vi "Estimate Posture from Velocity.vi"(8 "initialize":bool, 9 "dt (s)":dbl=1.0 format="%0.2f", 10 "initial posture":dbl[](array[numeric])=[0.0, 0.0, 0.0], 11 "estimated steering frame velocity":dbl[](array[numeric])=[0.0, 0.0, 0.0]) -> (3 "estimated steering frame posture":dbl[](array[numeric]))   [LabVIEW 2016]
doc: "This VI estimates the posture of a robot by integrating the measured velocity.\n\nThe velocity is a three element array consisting of lateral, forward, and angular velocities relative to the robot's frame of reference.\n\nThe posture is a three element array consiting of the X, Y, and angular position relative to a fixed global frame of reference."
uses:
  <vilib>/Analysis/coordinate.llb/Angle Range (Degree).ctl
  <vilib>/Analysis/coordinate.llb/Angle Units.ctl
  <vilib>/Analysis/coordinate.llb/Wrap Angle (scalar).vi
  <vilib>/Analysis/coordinate.llb/2D Cartesian Coordinate Rotation (Scalar).vi
  <vilib>/ptbypt/NI_PtbyPt.lvlib
  <vilib>/Analysis/NI_AALPro.lvlib
  <vilib>/Analysis/NI_AAL_Angle.lvlib
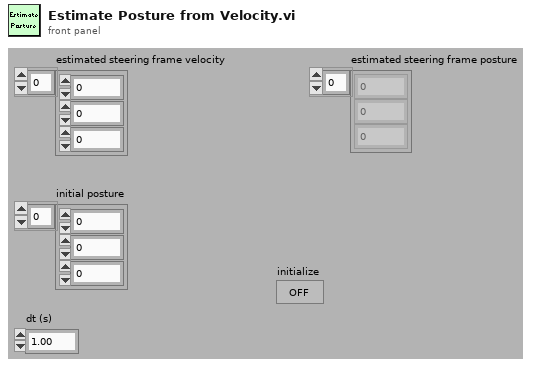
[diagram p1: front panel]
types:
  T1 = typedef "NI_AAL_Angle.lvlib/Angle Units.ctl" = i32
  T2 = typedef "NI_AAL_Angle.lvlib/Angle Range (Degree).ctl" = u16
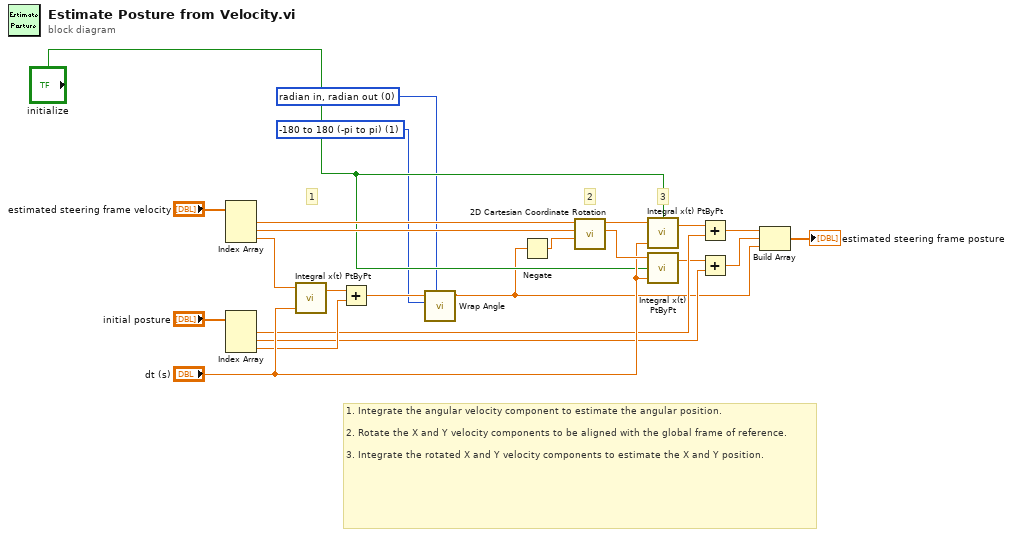
[diagram p0: block diagram]
diagram:
  w1 = T1 0 items=["radian in, radian out", "radian in, degree out", "degree in, degree out", "degree in, radian out"] ("angle units")
  w2 = T2 1 items=["none", "-180 to 180 (-pi to pi)", "0 to 360 (0 to 2pi)"] ("angle range")
  # "3"
  # "2"
  # "1. Integrate the angular velocity component to estimate the angular position.\n\n2. Rotate the X and Y velocity components to be aligned with the global frame of reference.\n\n3. Integrate the rotated X and Y velocity components to estimate the X and Y position."
  # "1"
  n1 = Index Array(array="estimated steering frame velocity") -> (element #1=w19:dbl, element #2=w18:dbl, element #3=w22:dbl)  [unwired: 3 in]
  n2 = Index Array(array="initial posture") -> (element #1=w11:dbl, element #2=w8:dbl, element #3=w13:dbl)  [unwired: 3 in]
  n3 = call <vilib>:"Integral x(t) PtByPt.vi"("dt"="dt (s)", "x"=w22) -> ("integral x(t)"=w12:dbl)  [unwired: 2 in, 1 out]
  n4 = Add(x=w12, y=w13) -> (x+y=w3:dbl)
  n5 = call-poly <vilib>:"Wrap Angle.vi"("angle units"=w1, "angle range"=w2, "angle in"=w3) -> ("angle out"=w4:dbl)  [unwired: 7 in, 1 out]
  n6 = Negate(x=w4) -> (-x=w20:dbl)
  n7 = call-poly <vilib>:"2D Cartesian Coordinate Rotation.vi"("theta"=w20, "y"=w18, "x"=w19) -> ("y out"=w16:dbl, "x out"=w17:dbl)  [unwired: 6 in, 1 out]
  n8 = call <vilib>:"Integral x(t) PtByPt.vi"("initialize"="initialize", "dt"="dt (s)", "x"=w17) -> ("integral x(t)"=w10:dbl)  [unwired: 1 in, 1 out]
  n9 = call <vilib>:"Integral x(t) PtByPt.vi"("initialize"="initialize", "dt"="dt (s)", "x"=w16) -> ("integral x(t)"=w7:dbl)  [unwired: 1 in, 1 out]
  n10 = Add(x=w10, y=w11) -> (x+y=w9:dbl)
  n11 = Add(x=w7, y=w8) -> (x+y=w6:dbl)
  n12 = Build Array(w9, w6, w4) -> (→"estimated steering frame posture":dbl[])
